vi "Add Caption and image V2.vi"(0 "PDF Report IN":refnum<class "PDF Report Class.lvclass">, 2 "Caption?":bool, 5 "Paragraph Refnum":refnum<k24>, 9 "Image Ref iTexSharp":refnum<k24>, 11 "error in (no error)":errorcluster) -> (4 "PDF Report OUT":refnum<class "PDF Report Class.lvclass">, 8 "Size (points)":cluster{"TotalHeight":sgl, "TotalWidth":sgl}, 15 "error out":errorcluster)   [LabVIEW 2019]
doc: "Version 1.0\nDeveloped by Jean-Marc Simard\nCopyright © 2010, Exaprom Inc.\nAll rights reserved.\nLicense: BSD\n\nWith iTextSharp 4.1.6 (http://itextsharp.sourceforge.net)\nunder Mozilla Public License Version 1.1\n(http://www.mozilla.org/MPL/MPL-1.1.html)"
uses:
  <userlib>/Exaprom PDF/LV Class/PDF Report Class/PDF Report Class.lvclass
  C:/Program Files/National Instruments/LabVIEW 2019/user.lib/Exaprom PDF/DLL/itextsharp.dll
  DLL/itextsharp.dll
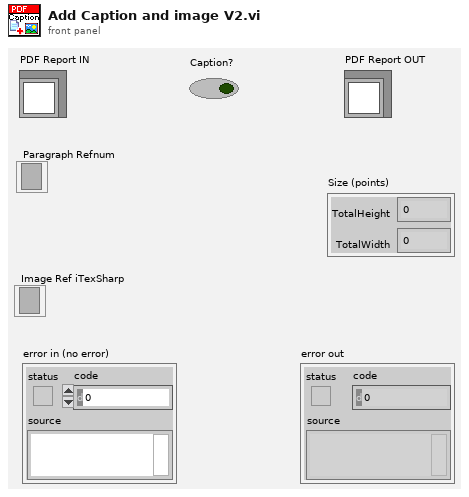
[diagram p1: front panel]
types:
  T1 = typedef "Captions.ctl" = cluster{"Figure":T2, "Table":T2, "Font":T3}
  T2 = typedef "Image or Table Caption.ctl" = cluster{"Caption":string, "Separator":string, "Position":enum16{"Above", "Below"}}
  T3 = typedef "Font complete cluster.ctl" = cluster{"Name":string, "Size":T4, "Color":T5, "Style":cluster{"Bold":bool, "Italic":bool, "Underline":bool, "Strikeout":bool}, "Type":T6}
  T4 = typedef "Font size.ctl" = sgl
  T5 = typedef "Font color.ctl" = u32
  T6 = typedef "Type and encoding.ctl" = cluster{"Type&direction":T7, "Embedded":bool, "Encoding":string}
  T7 = typedef "Type and run direction.ctl" = enum16{"Select", "ASCII", "UTF-16", "UTF-16 (default)", "UTF-16 (LTR)", "UTF-16 (RTL)"}
  T8 = cluster{"Captions":T1, "Image counter":u16, "Table counter":u16}
  T9 = typedef "Page dimensions.ctl" = cluster{"Start at page":i32, "Page Size":T10, "Orientation":T11, "widht":sgl, "height":sgl, "Margin left":sgl, "Margin right":sgl, "Margin top":sgl, "Margin bottom":sgl, "X0":sgl, "X1":sgl, "Y0":sgl, "Y1":sgl}
  T10 = typedef "Page size.ctl" = i32
  T11 = typedef "Page Orientation.ctl" = enum16{"Portrait", "Landscape"}
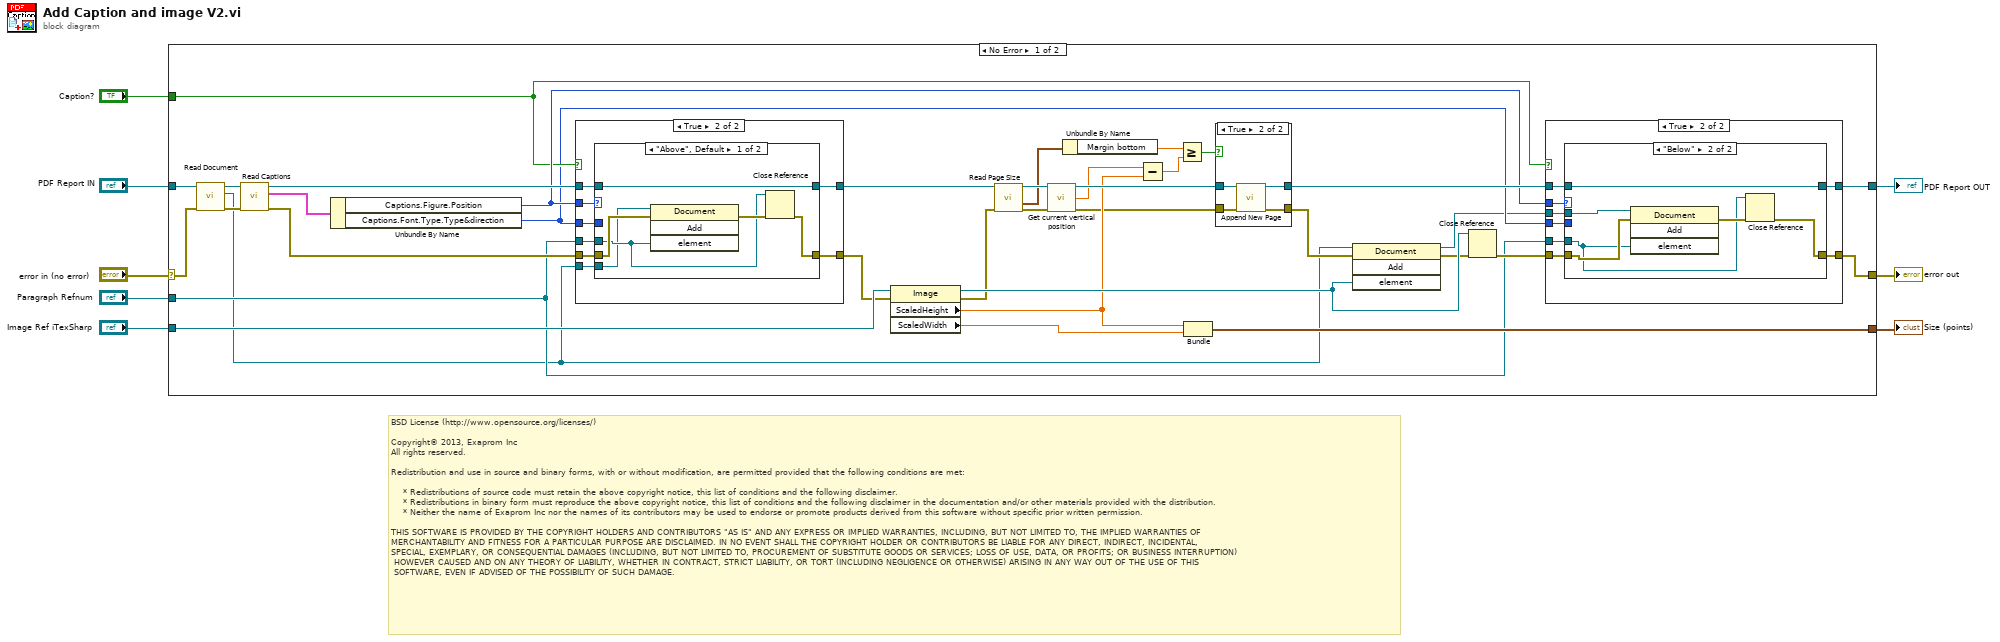
[diagram p0: block diagram]
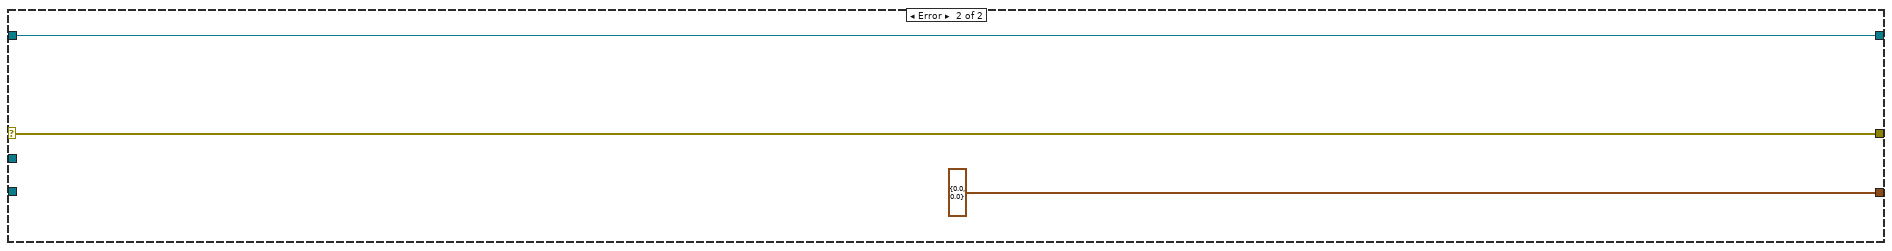
[diagram p7: hidden frame]
diagram:
  # "BSD License (http://www.opensource.org/licenses/)\n\nCopyright© 2013, Exaprom Inc\nAll rights reserved.\n\nRedistribution and use in source and binary forms, with or without modification, are permitted provided that the following conditions are met:\n\n    * Redistributions of source code must retain the above copyright notice, this list of conditions and the following disclaimer.\n    * Redistributions in binary form must reproduce the above copyright notice, this list of conditions and the following disclaimer in the documentation and/or other materials provided with the distribution.\n    * Neither the name of Exaprom Inc nor the names of its contributors may be used to endorse or promote products derived from this software without specific prior written permission.\n\nTHIS SOFTWARE IS PROVIDED BY THE COPYRIGHT HOLDERS AND CONTRIBUTORS \"AS IS\" AND ANY EXPRESS OR IMPLIED WARRANTIES, INCLUDING, BUT NOT LIMITED TO, THE IMPLIED WARRANTIES OF \nMERCHANTABILITY AND FITNESS FOR A PARTICULAR PURPOSE ARE DISCLAIMED. IN NO EVENT SHALL THE COPYRIGHT HOLDER OR CONTRIBUTORS BE LIABLE FOR ANY DIRECT, INDIRECT, INCIDENTAL,\nSPECIAL, EXEMPLARY, OR CONSEQUENTIAL DAMAGES (INCLUDING, BUT NOT LIMITED TO, PROCUREMENT OF SUBSTITUTE GOODS OR SERVICES; LOSS OF USE, DATA, OR PROFITS; OR BUSINESS INTERRUPTION)\n HOWEVER CAUSED AND ON ANY THEORY OF LIABILITY, WHETHER IN CONTRACT, STRICT LIABILITY, OR TORT (INCLUDING NEGLIGENCE OR OTHERWISE) ARISING IN ANY WAY OUT OF THE USE OF THIS\n SOFTWARE, EVEN IF ADVISED OF THE POSSIBILITY OF SUCH DAMAGE."
  n1 = case shown="No Error" "error in (no error)" {
    selector: "error in (no error)" -> [w22 w89]
    tunnel: "PDF Report IN" -> [w43 w88]
    tunnel: [w17 w88] -> w7
    tunnel: [w15 w89] -> w6
    tunnel: [w44 cluster{"ScaledHeight":sgl, "ScaledWidth":sgl} {"ScaledHeight"=0.0, "ScaledWidth"=0.0}] -> w3
    tunnel: "Image Ref iTexSharp" -> [w42 _]
    tunnel: "Caption?" -> [w13 _]
    tunnel: "Paragraph Refnum" -> [w12 _]
    frame No Error {
      n2 = call-dynamic "Read Document.vi"("error in (no error)"=w22, "PDF Report Class in"=w43) -> ("error out"=w23:errorcluster, "Document"=w10:refnum<k24>, "PDF Report Class out"=w25:refnum<class "PDF Report Class.lvclass">)  [unwired: 7 in]
      n3 = call-dynamic "Read Captions.vi"("error in (no error)"=w23, "PDF Report Class in"=w25) -> ("error out"=w21:errorcluster, "Captions and counters"=w24:T8, "PDF Report Class out"=w20:refnum<class "PDF Report Class.lvclass">)  [unwired: 7 in]
      n4 = Unbundle By Name(w24) -> ("Captions.Figure.Position"=w14:enum16{"Above", "Below"}, "Captions.Font.Type.Type&direction"=w11:T7)
      n5 = case shown="True" w13 {
        tunnel: w21 -> [w64 w72]
        tunnel: [w64 w71] -> w26
        tunnel: w14 -> [_ w70]
        tunnel: w12 -> [_ w69]
        tunnel: w20 -> [w63 w68]
        tunnel: [w63 w67] -> w19
        tunnel: w11 -> [_ w66]
        tunnel: w10 -> [_ w65]
        frame False {
        }
        frame True {
          n6 = case shown="\"Above\", Default" w70 {
            tunnel: w69 -> [w74 _]
            tunnel: w72 -> [w76 w80]
            tunnel: [w75 w80] -> w71
            tunnel: w68 -> [w77 w79]
            tunnel: [w77 w79] -> w67
            tunnel: w66 -> [_ _]
            tunnel: w65 -> [w73 _]
            frame "Above", Default {
              n7 = invoke class="Document" method="Add"(reference=w73, error in=w76, "element"=w74) -> (error out=w78:errorcluster)  [unwired: 1 in, 3 out]
              n8 = Close Reference(reference=w74, error in (no error)=w78) -> (error out=w75:errorcluster)
            }
            frame "Below" {
            }
          }
        }
      }
      n9 = property class="Image"(reference=w42, error in=w26) -> (reference out=w41:refnum<k24>, error out=w32:errorcluster, "ScaledHeight"=w33:sgl, "ScaledWidth"=w40:sgl)
      n10 = call <userlib>:"Read Page Size.vi"("PDF Report"=w19, "error in (no error)"=w32) -> ("PDF Report duplicate"=w38:refnum<class "PDF Report Class.lvclass">, "Page (points)"=w36:T9, "error out"=w37:errorcluster)  [unwired: 11 out]
      n11 = call <userlib>:"Get current vertical position.vi"("PDF Report In"=w38, "error in (no error)"=w37) -> ("PDF Report duplicate"=w39:refnum<class "PDF Report Class.lvclass">, "GetVerticalPosition (points)"=w34:sgl, "error out"=w29:errorcluster)  [unwired: 1 in, 10 out]
      n12 = Unbundle By Name(w36) -> ("Margin bottom"=w35:sgl)
      n13 = Subtract(x=w34, y=w33) -> (x-y=w31:sgl)
      n14 = Greater Or Equal?(x=w35, y=w31) -> (x >= y?=w30:bool)
      n15 = Bundle("ScaledHeight"=w33, "ScaledWidth"=w40) -> (w44:cluster{"ScaledHeight":sgl, "ScaledWidth":sgl})  [unwired: 1 out]
      n16 = case shown="True" w30 {
        tunnel: w39 -> [w82 w86]
        tunnel: [w82 w85] -> w18
        tunnel: w29 -> [w81 w84]
        tunnel: [w81 w83] -> w28
        frame False {
        }
        frame True {
          n17 = call <userlib>:"Append New Page.vi"("PDF Report"=w86, "error in (no error)"=w84) -> ("PDF Report duplicate"=w85:refnum<class "PDF Report Class.lvclass">, "error OUT"=w83:errorcluster)  [unwired: 12 out]
        }
      }
      n18 = invoke class="Document" method="Add"(reference=w10, error in=w28, "element"=w41) -> (reference out=w9:refnum<k24>, error out=w27:errorcluster)  [unwired: 1 in, 2 out]
      n19 = Close Reference(reference=w41, error in (no error)=w27) -> (error out=w16:errorcluster)
      n20 = case shown="True" w13 {
        tunnel: w16 -> [w46 w54]
        tunnel: [w46 w53] -> w15
        tunnel: w14 -> [_ w52]
        tunnel: w12 -> [_ w51]
        tunnel: w18 -> [w45 w50]
        tunnel: [w45 w49] -> w17
        tunnel: w11 -> [_ w48]
        tunnel: w9 -> [_ w47]
        frame False {
        }
        frame True {
          n21 = case shown="\"Below\"" w52 {
            tunnel: w51 -> [_ w57]
            tunnel: w54 -> [w56 w58]
            tunnel: [w56 w60] -> w53
            tunnel: w50 -> [w55 w61]
            tunnel: [w55 w61] -> w49
            tunnel: w48 -> [_ _]
            tunnel: w47 -> [_ w59]
            frame "Above", Default {
            }
            frame "Below" {
              n22 = invoke class="Document" method="Add"(reference=w59, error in=w58, "element"=w57) -> (error out=w62:errorcluster)  [unwired: 1 in, 3 out]
              n23 = Close Reference(reference=w57, error in (no error)=w62) -> (error out=w60:errorcluster)
            }
          }
        }
      }
    }
    frame Error {
    }
  }
  "PDF Report OUT" <- w7
  "error out" <- w6
  "Size (points)" <- w3
